vi "PROG 8 - CONVERSION OF TEMPERATURE USING FORMULA NODE BY TAKING INPUT AND DISPLAY OUTPUT.vi"() -> ()   [LabVIEW 2012]
panel:
  out "THE TEMPERATURE IN CELSIUS IS:":dbl
  in  "ENTER TEMPERATURE IN DEGREE FAHRENHEIT":dbl
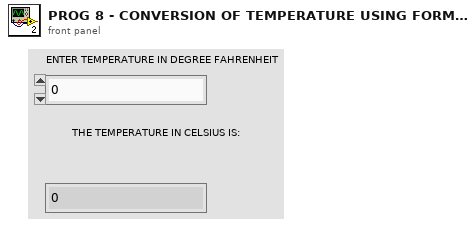
[diagram p1: front panel]
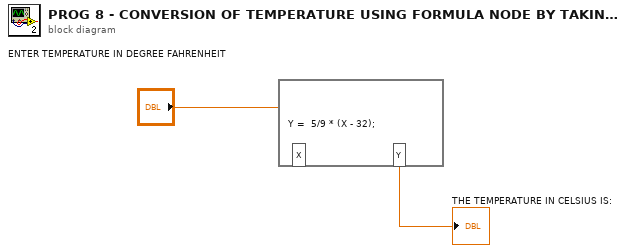
[diagram p0: block diagram]
diagram:
  n1 = formula code="Y =  5/9 * (X - 32);"("X"="ENTER TEMPERATURE IN DEGREE FAHRENHEIT") -> ("Y"=→"THE TEMPERATURE IN CELSIUS IS:":dbl)
